vi "Read-LVDT-Data.vi"(0 "shared variable refnum":refnum<k21>, 2 "MaxLen":i32, 9 "Data IN":dbl[](array[numeric])) -> (4 "Graph Data":dbl[](array[numeric]), 10 "Data OUT":dbl[](array[numeric]), 15 "error out":errorcluster)   [LabVIEW 2011]
uses:
  <vilib>/Analysis/6fits.llb/Remove Outliers (Range).vi
  <vilib>/Analysis/NI_AALPro.lvlib
panel:
  out "size(s)":i32
  out "Outlier Indexes":i32[](array[numeric])
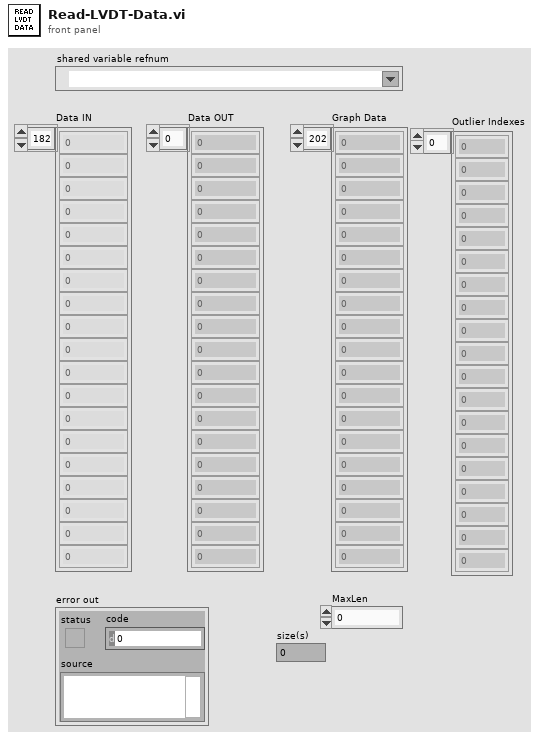
[diagram p1: front panel]
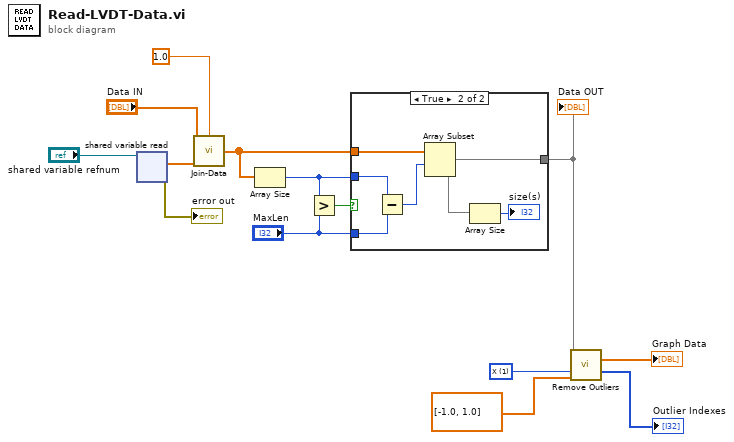
[diagram p0: block diagram]
diagram:
  w8 = u16 1 items=["Y", "X", "X and Y"] ("range type")
  n1 = shared-variable-read("shared variable refnum") -> (→"error out":errorcluster, w12:dbl[])  [unwired: 1 in, 2 out]
  n2 = call "Join-Data.vi"("Existing Data"="Data IN", "threshold"=1.0, "New Data"=w12) -> ("Output"=w5:dbl[])  [unwired: 12 in]
  n3 = Array Size(array=w5) -> (size(s)=w2:i32)
  n4 = Greater?(x=w2, y="MaxLen") -> (0:w4:bool)
  n5 = case shown="True" w4 {
    tunnel: w5 -> [w15 w21]
    tunnel: [w15 w17] -> w3
    tunnel: w2 -> [_ w20]
    tunnel: "MaxLen" -> [_ w19]
    frame False {
    }
    frame True {
      n6 = Subtract(x=w20, y=w19) -> (x-y=w18:i32)
      n7 = Array Subset(array=w21, index=w18) -> (w17:dbl[])  [unwired: 1 in]
      n8 = Array Size(array=w17) -> (size(s)=→"size(s)":i32)
    }
  }
  "Data OUT" <- w3
  n9 = call-poly <vilib>:"Remove Outliers.vi"("Y"=w3, "X"=w3, "range type"=w8, "Range"=dbl[] [-1.0, 1.0]) -> ("X Out"=→"Graph Data":dbl[], "Outlier Indexes"=→"Outlier Indexes":i32[])  [unwired: 7 in, 3 out]
